vi "clean_up_in_loop (SubVI).vi"(11 "Refnum in":refnum<k21>) -> (3 "Refnum out":refnum<k21>)   [LabVIEW 2016]
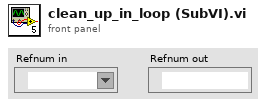
[diagram p1: front panel]
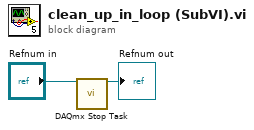
[diagram p0: block diagram]
diagram:
  n1 = call <vilib>:"DAQmx Stop Task.vi"("task/channels in"="Refnum in") -> ("task out"=→"Refnum out":refnum<k21>)  [unwired: 13 in, 1 out]
